vi "Select All Items.vi"(0 "Display State In":T1, 9 "Container State":T2, 11 "error in (no error)":errorcluster) -> (4 "Display State Out":T1, 15 "error out":errorcluster)   [LabVIEW 2014, in "ListBox XControl.xctl"]
uses:
  ListBox XControl.xctl
  <vilib>/_xctls/Container State.ctl
  State ListBox.ctl
  <vilib>/_xctls/XControlSupport.lvlib
panel:
  # "Add Controls & Indicators that form the parameters of the method here. Hook them to the connector pane. Do not delete the controls & indicators that are already hooked to the connector pane.\n \nTo setup the parameters  for this method, right click on this item in the Project Tree & select \"Configure Method...\"."
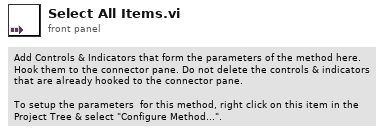
[diagram p1: front panel]
types:
  T1 = typedef "ListBox XControl.xctl/State ListBox.ctl" = cluster{"ItemNames[]":string[], "Listbox Ref":refnum<vi>, "Select All By Default":bool}
  T2 = typedef "XControlSupport.lvlib/Container State.ctl" = cluster{"Indicator?":bool, "Run Mode?":bool, " Refnum":refnum<vi>}
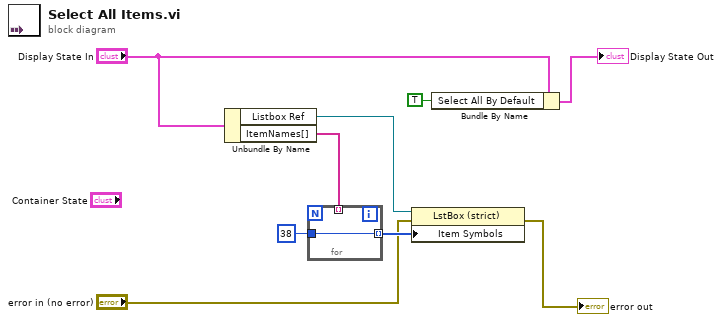
[diagram p0: block diagram]
diagram:
  n1 = Unbundle By Name("Display State In") -> ("Listbox Ref"=w9:refnum<vi>, "ItemNames[]"=w8:string[])
  n2 = for {
    tunnel: w8 -> [_] mode=indexing
    tunnel: [w10] -> w7 mode=indexing
    tunnel: 38 -> [w10]
  }
  n3 = property class="LstBox (strict)"(reference=w9, error in="error in (no error)", "Item Symbols"=w7) -> (error out=→"error out":errorcluster)  [unwired: 1 out]
  n4 = Bundle By Name(cluster="Display State In", "Select All By Default"=TRUE) -> (→"Display State Out":T1)
